vi "Freqsync.vi"(1 "Frequency Offset":dbl, 2 "Offset Signal 2":cdb[](array[numeric])) -> (0 "Corrected Signal 2":cdb[](array[numeric]))   [LabVIEW 2013]
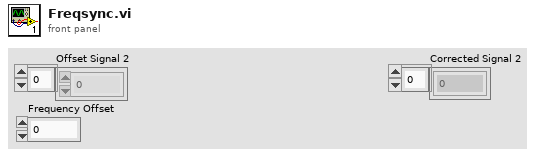
[diagram p1: front panel]
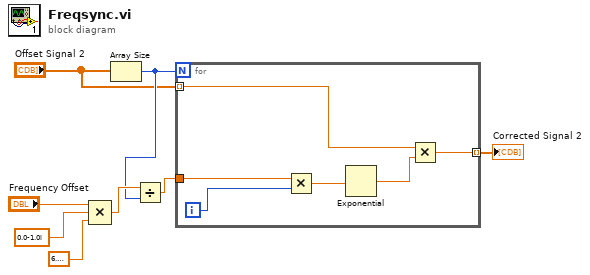
[diagram p0: block diagram]
diagram:
  n1 = Compound Arithmetic op=MULTIPLY("Frequency Offset", cdb 0.0-1.0i ("value"), 6.283185307179586) -> (w4:cdb)
  n2 = Array Size(array="Offset Signal 2") -> (size(s)=w3:i32)
  n3 = Divide(x=w4, y=w3) -> (x/y=w1:cdb)
  n4 = for {
    N: w3 -> [_]
    tunnel: [w14] -> w8 mode=indexing
    tunnel: "Offset Signal 2" -> [w13] mode=indexing
    tunnel: w1 -> [w9]
    i -> [w10]
    n5 = Multiply(x=w9, y=w10) -> (x*y=w11:cdb)
    n6 = Exponential(1:w11) -> (0:w12:cdb)
    n7 = Multiply(x=w13, y=w12) -> (x*y=w14:cdb)
  }
  "Corrected Signal 2" <- w8
